vi "Insert Menu Items (if not exist).vi"(6 "after item":string, 7 "menu tag":string, 8 "error in (no error)":errorcluster, 9 "item tag":string, 10 "item name":string, 11 "Menu in":refnum<k9>) -> (0 "error out":errorcluster, 1 "tag out":string, 3 "Menu out":refnum<k9>)   [LabVIEW 2019, in "Menu From Cluster.lvlib"]
uses:
  Menu From Cluster.lvlib
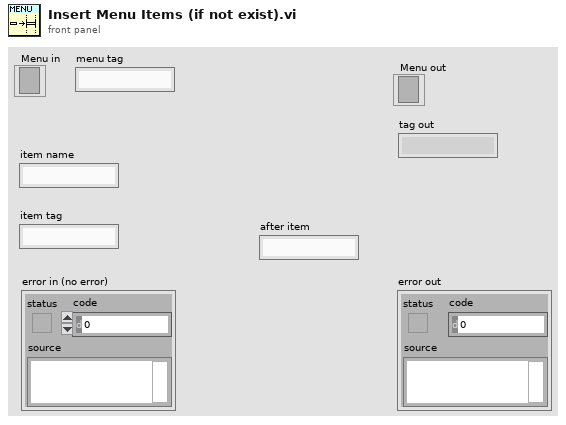
[diagram p1: front panel]
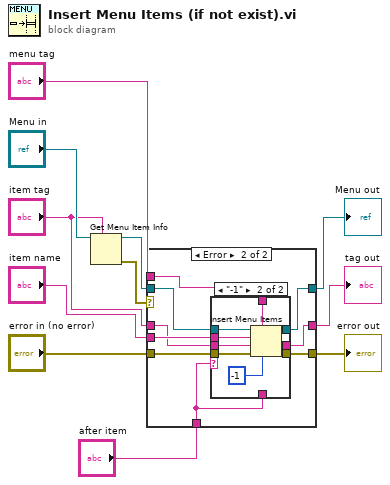
[diagram p0: block diagram]
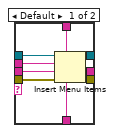
[diagram p3: hidden frame]
diagram:
  n1 = Get Menu Item Info(7:"item tag", 11:"Menu in") -> (0:w2:errorcluster, 3:w3:refnum<k9>)  [unwired: 1 in, 5 out]
  n2 = case shown="Error" w2 {
    tunnel: "item name" -> [_ w23]
    tunnel: [w13 w22] -> w10
    tunnel: "menu tag" -> [_ w21]
    tunnel: "error in (no error)" -> [w12 w20]
    tunnel: [w14 w19] -> w7
    tunnel: [w12 w18] -> w6
    tunnel: "item tag" -> [w13 w17]
    tunnel: w3 -> [w14 w16]
    tunnel: "after item" -> [_ w15]
    frame No Error {
      # "Already exists"
    }
    frame Error {
      n3 = case shown="\"-1\"" w15 {
        tunnel: w23 -> [w32 w41]
        tunnel: [w31 w40] -> w22
        tunnel: w21 -> [w30 w39]
        tunnel: w20 -> [w29 w38]
        tunnel: [w28 w37] -> w19
        tunnel: [w27 w36] -> w18
        tunnel: w17 -> [w26 w35]
        tunnel: w16 -> [w25 w34]
        tunnel: w15 -> [w24 _]
        frame Default {
          n4 = Insert Menu Items(4:w24, 5:w30, 6:w29, 7:w26, 8:w32, 9:w25) -> (0:w27:errorcluster, 1:w31:string, 3:w28:refnum<k9>)
        }
        frame "-1" {
          n5 = Insert Menu Items(4:-1, 5:w39, 6:w38, 7:w35, 8:w41, 9:w34) -> (0:w36:errorcluster, 1:w40:string, 3:w37:refnum<k9>)
        }
      }
    }
  }
  "tag out" <- w10
  "Menu out" <- w7
  "error out" <- w6
